vi "Main.vi"() -> ()   [LabVIEW 2017]
uses:
  logo.ctl
  <vilib>/Utility/error.llb/DialogType.ctl
  <userlib>/SimuLabAPIEx_V3/SimuLabAPIEx_V3.lvlib
panel:
  out "剩余日志条数":i32
  out "function return 2":i32
  out "nStatus out":i32
  out "注册参数瞬态返回值":i32
  in  "信号1":i32(listbox)
  out "方法返回值":i32
  in  "注销录制组":bool
  in  "录制组名称":string
  out "录制组状态":i32
  out "方法返回值":i32
  in  "获取录制组状态":bool
  in  "录制组名称":string
  in  "列表长度":i32
  out "方法返回值":i32
  out "返回信号ID":i32
  in  "获取信号ID通过名称":bool
  in  "信号名称":string
  out "function return":i32
  out "nOutSigParamOffsetList out":i32[](array[numeric])
  out "nOutSigParamIdList out":i32[](array[numeric])
  in  "注册录制组":bool
  in  "参数输出信号偏移":i32[](array[numeric])
  in  "参数/输出信号ID列表":i32[](array[numeric])
  in  "录制文件名":string
  in  "存储文件的路径":string
  in  "数据格式":i32
  in  "录制时长":dbl
  in  "采样率":i32
  in  "录制组名称":string
  out "信号连续返回值":dbl[](array[numeric])
  out "pTimeOffset out":dbl[](array[numeric])
  out "实际有效数据长度":i32
  out "信连方法返回值":i32
  in  "获取信号值连续":bool
  in  "数组偏移":i32
  in  "信号名称":string
  out "返回的信号值":dbl[](array[numeric])
  out "实际有效数据长度":i32
  out "时间偏移返回值":dbl
  out "信瞬方法返回值":i32
  in  "获取信号值瞬态":bool
  in  "数组偏移":i32
  in  "信号名称":string
  out "方法返回值":i32
  out "返回的日志级别":i32
  out "返回的日志信息":string
  out "返回的时间偏移":dbl[](array[numeric])
  out "返回的参数值":dbl[](array[numeric])
  out "实际有效数据长度":i32
  out "获取参数值连续返回值":i32
  in  "获取参数值连续":bool
  in  "数组偏移":i32
  in  "参数名称":string
  out "实际有效数据长度":i32
  out "时间偏移返回值":dbl
  out "pDataValue out":dbl[](array[numeric])
  out "获取参数值瞬态返回值":i32
  in  "获取参数值瞬态":bool
  in  "数组偏移":i32
  in  "参数名称":string
  out "注销输出信号连续返回值":i32
  in  "注销输出信号连续":bool
  in  "数组偏移":i32
  in  "输出信号名称":string
  out "注册输出信号连续返回值":i32
  in  "注册输出信号连续":bool
  in  "数组偏移":i32
  in  "输出信号名称":string
  out "注销输出信号瞬态返回值":i32
  in  "注销输出信号瞬态":bool
  in  "数组偏移":i32
  in  "输出信号名称":string
  out "注册输出信号瞬态返回值":i32
  in  "注册输出信号瞬态":bool
  in  "数组偏移":i32
  in  "输出信号名称":string
  out "pData":dbl[](array[numeric])
  out "方法返回值":i32
  in  "获取参数值":bool
  in  "数组偏移量":i32
  in  "参数名称":string
  out "注销连续返回值":i32
  in  "注销连续":bool
  in  "数组偏移":i32
  in  "参数名称":string
  out "注册参数连续返回值":i32
  in  "注册参数连续":bool
  in  "数组偏移":i32
  in  "参数名称":string
  out "注销参数瞬态返回值":i32
  in  "注销参数瞬态":bool
  in  "数组偏移":i32
  in  "参数名称":string
  in  "数组偏移":i32
  in  "注册参数瞬态":bool
  in  "参数名称":string
  in  "数组偏移量":i32
  out "pData":dbl[](array[numeric])
  out "方法返回值":i32
  in  "获取信号值":bool
  in  "信号名称":string
  out "方法返回值":i32
  out "模型名称":string
  in  "根据参数名称获取模型名称":bool
  in  "参数名称":string
  out "方法返回值":i32
  out "返回参数ID":i32
  in  "获取参数ID通过名称":bool
  in  "参数名称":string
  out "方法返回值":i32
  out "返回模型ID":i32
  in  "模型名称获取ID":bool
  in  "模型名称":string
  out "返回的下位机IP":string
  in  "模型的下位机IP":bool
  in  "模型名称":string
  out "方法返回值":i32
  out "返回的模型信息":string
  in  "获取指定模型序号模型信息":bool
  in  "模型序号":i32
  out "参数个数":i32
  in  "获取参数个数":bool
  out "模型个数":i32
  in  "获取模型个数":bool
  in  "获取仿真系统日志信息":bool
  out "dMoniData":dbl[](array[numeric])
  out "超时返回值":i32
  out "方法返回值":i32
  in  "获取模型仿真状态":bool
  in  "模型名称输入框":string
  out "方法返回值":i32
  out "状态返回值":i32
  in  "获取工程状态":bool
  out "方法返回值":i32
  out "返回的错误信息":string
  in  "获取最后错误信息":bool
  in  "缓冲点数":i32=20000
  in  "参数索引（1-N）":i32=1 min=1
  in  "缓冲示波个数":i32=10000
  in  "列表已更新":bool=TRUE
  in  "刷新图形":bool
  out "XY Graph":T1(graph)={"pTimeOffset out"=[747.164, 747.165, 747.166, 747.167, 747.168, 747.169, 747.17, 747.171, 747.172, 747.173, 747.174, 747.1750000000001, 747.176, 747.177, 747.178, 747.179, 747.1800000000001, 747.181, 747.182, 747.183, 747.184, 747.1850000000001, 747.186, 747.187, 747.188, 747.189, 747.19, 747.191, 747.192, 747.193, 747.194, 747.195, 747.196, 747.197, 747.198, 747.1990000000001, 747.2, 747.201, 747.202, 747.203, 747.2040000000001, 747.205, 747.206, 747.207, 747.208, 747.2090000000001, 747.21, 747.211, 747.212, 747.213, 747.214, 747.215, 747.216, 747.217, 747.218, 747.219, 747.22, 747.221, 747.222, 747.2230000000001, 747.224, 747.225, 747.226, 747.227, 747.2280000000001, 747.229, 747.23, 747.231, 747.232, 747.2330000000001, 747.234, 747.235, 747.236, 747.237, 747.238, 747.239, 747.24, 747.241, 747.242, 747.243, 747.244, 747.245, 747.246, 747.2470000000001, 747.248, 747.249, 747.25, 747.251, 747.2520000000001, 747.253, 747.254, 747.255, 747.256, 747.2570000000001, 747.258, 747.259, 747.26, 747.261, 747.2620000000001, 747.263, 747.264, 747.265, 747.266, 747.267, 747.268, 747.269, 747.27, 747.2710000000001, 747.272, 747.273, 747.274, 747.275, 747.2760000000001, 747.277, 747.278, 747.279, 747.28, 747.2810000000001, 747.282, 747.283, 747.284, 747.285, 747.2860000000001, 747.287, 747.288, 747.289, 747.29, 747.291, 747.292, 747.293, 747.294, 747.295, 747.296, 747.297, 747.298, 747.299, 747.3000000000001, 747.301, 747.302, 747.303, 747.304, 747.3050000000001, 747.306, 747.307, 747.308, 747.309, 747.3100000000001, 747.311, 747.312, 747.313, 747.314, 747.315, 747.316, 747.317, 747.318, 747.319, 747.32, 747.321, 747.322, 747.323, 747.3240000000001, 747.325, 747.326, 747.327, 747.328, 747.3290000000001, 747.33, 747.331, 747.332, 747.333, 747.3340000000001, 747.335, 747.336, 747.337, 747.338, 747.339, 747.34, 747.341, 747.342, 747.343, 747.344, 747.345, 747.346, 747.347, 747.3480000000001, 747.349, 747.35, 747.351, 747.352, 747.3530000000001, 747.354, 747.355, 747.356, 747.357, 747.3580000000001, 747.359, 747.36, 747.361, 747.362, 747.363, 747.364, 747.365, 747.366, 747.367, 747.368, 747.369, 747.37, 747.371, 747.3720000000001, 747.373, 747.374, 747.375], "pDataValue out"=[-0.5107453766165692, -0.509885389359039, -0.5090248922161622, -0.5081638860483376, -0.5073023717167672, -0.5064403500828674, -0.5055778220086596, -0.5047147883566722, -0.5038512499898401, -0.5029872077718983, -0.5021226625667906, -0.5012576152390622, -0.500392066653662, -0.4995260176763352, -0.49865946917303233, -0.49779242201030194, -0.496924877055191, -0.4960568351751457, -0.4951882972384053, -0.49431926411340893, -0.4934497366691897, -0.4925797157752749, -0.4917092023015864, -0.49083819711883553, -0.4899667010979285, -0.4890947151103612, -0.4882222400281196, -0.48734927672357936, -0.48647582606990225, -0.48560188894043965, -0.48472746620912865, -0.4838525587503918, -0.482977167439037, -0.48210129315065453, -0.48122493676101913, -0.4803480991464871, -0.47947078118379616, -0.4785929837504638, -0.4777147077241875, -0.47683595398324335, -0.475956723406385, -0.47507701687274284, -0.47419683526222345, -0.47331617945490834, -0.4724350503314532, -0.47155344877298716, -0.4706713756610113, -0.46978883187779935, -0.46890581830579464, -0.4680223358280108, -0.46713838532793006, -0.4662539676894024, -0.46536908379704645, -0.4644837345356455, -0.4635979207905488, -0.4627116434475699, -0.46182490339288534, -0.46093770151343666, -0.4600500386963249, -0.4591619158292128, -0.4582733338001221, -0.45738429349783677, -0.45649479581129615, -0.45560484162999776, -0.4547144318438957, -0.45382356734329843, -0.4529322490192729, -0.45204047776303613, -0.4511482544663593, -0.4502555800214656, -0.44936245532092783, -0.44846888125807377, -0.4475748587263758, -0.4466803886198565, -0.4457854718329857, -0.44489010926057854, -0.44399430179820093, -0.4430980503415586, -0.4422013557869028, -0.4413042190309281, -0.44040664097066906, -0.4395086225039079, -0.4386101645285608, -0.43771126794308574, -0.43681193364627696, -0.4359121625376732, -0.43501195551694327, -0.43411131348429405, -0.43321023734036757, -0.43230872798613734, -0.43140678632331764, -0.4305044132537476, -0.42960160967980016, -0.4286983765042789, -0.42779471463031415, -0.4268906249617731, -0.42598610840264267, -0.4250811658574394, -0.4241757982311057, -0.42327000642890616, -0.4223637913568384, -0.4214571539210145, -0.42055009502807184, -0.4196426155850692, -0.41873471649938276, -0.4178263986791179, -0.41691766303248917, -0.41600851046823223, -0.41509894189539603, -0.41418895822375595, -0.4132785603631922, -0.4123677492241025, -0.411456525717298, -0.41054489075389844, -0.40963284524574595, -0.40872039010478234, -0.4078075262434627, -0.4068942545746509, -0.4059805760115145, -0.4050664914679398, -0.4041520018579074, -0.40323710809590685, -0.40232181109683185, -0.40140611177587515, -0.4004900110489442, -0.3995735098320356, -0.3986566090416505, -0.3977393095946896, -0.3968216124083479, -0.39590351840053123, -0.3949850284892291, -0.39406614359293146, -0.3931468646305231, -0.39222719252117827, -0.3913071281847782, -0.39038667254128256, -0.3894658265111469, -0.38854459101511246, -0.3876229669746241, -0.38670095531120113, -0.3857785569468551, -0.38485577280398425, -0.3839326038052677, -0.3830090508740843, -0.382085114933882, -0.38116079690859656, -0.380236097722546, -0.37931101830032427, -0.37838555956722103, -0.3774597224485897, -0.37653350787026746, -0.37560691675846875, -0.37467995003967913, -0.3737526086410761, -0.3728248934898956, -0.37189680551385274, -0.3709683456410353, -0.3700395147997976, -0.3691103139191815, -0.36818074392828226, -0.3672508057566698, -0.3663205003341764, -0.36538982859131897, -0.3644587914586634, -0.36352738986724675, -0.36259562474847057, -0.36166349703399386, -0.36073100765615623, -0.359798157547341, -0.3588649476403983, -0.3579313788685378, -0.3569974521652221, -0.3560631684645902, -0.35512852870081946, -0.3541935338085497, -0.3532581847227756, -0.35232248237873987, -0.3513864277123575, -0.35045002165957667, -0.3495132651568035, -0.3485761591407942, -0.3476387045485483, -0.3467009023177334, -0.345762753386045, -0.34482425869163214, -0.3438854191728825, -0.34294623576884914, -0.3420067094186086, -0.34106684106168716, -0.3401266316379531, -0.3391860820875088, -0.33824519335111763, -0.3373039663695613, -0.3363624020840667, -0.33542050143619806, -0.33447826536774883, -0.33353569482116924, -0.3325927907389226, -0.33164955406391294, -0.33070598573937693, -0.3297620867087754, -0.3288178579162219, -0.327873300305838, -0.32692841482218105, -0.32598320241013656, -0.3250376640148094, -0.3240918005819527, -0.3231456130573225, -0.32219910238710614, -0.32125226951770663, -0.320305115396172, -0.31935764096954866]} caption="信号波形图"
  in  "工程配置文件":path=path "C:/testProj/testProj/main.slm"
  out "加载状态":bool
  out "加载返回值":i32 caption="返回值"
  in  "参数":i32(listbox)=-1
  in  "信号":i32(listbox)=2
  in  "重置":bool
  in  "暂停":bool
  in  "开始":bool
  in  "加载":bool
  in  "logo":T2
  in  "退出":bool
  out "连接状态":bool=TRUE
  out "连接返回值":i32 caption="返回值"
  in  "仿真系统上位机IP地址":string="192.168.1.52"
  in  "连接":bool
  # "Simulab 仿 真 测 试 平 台 演 示 Demo V3.0"
  # "双击参数进行调参"
  # "双击信号图形显示"
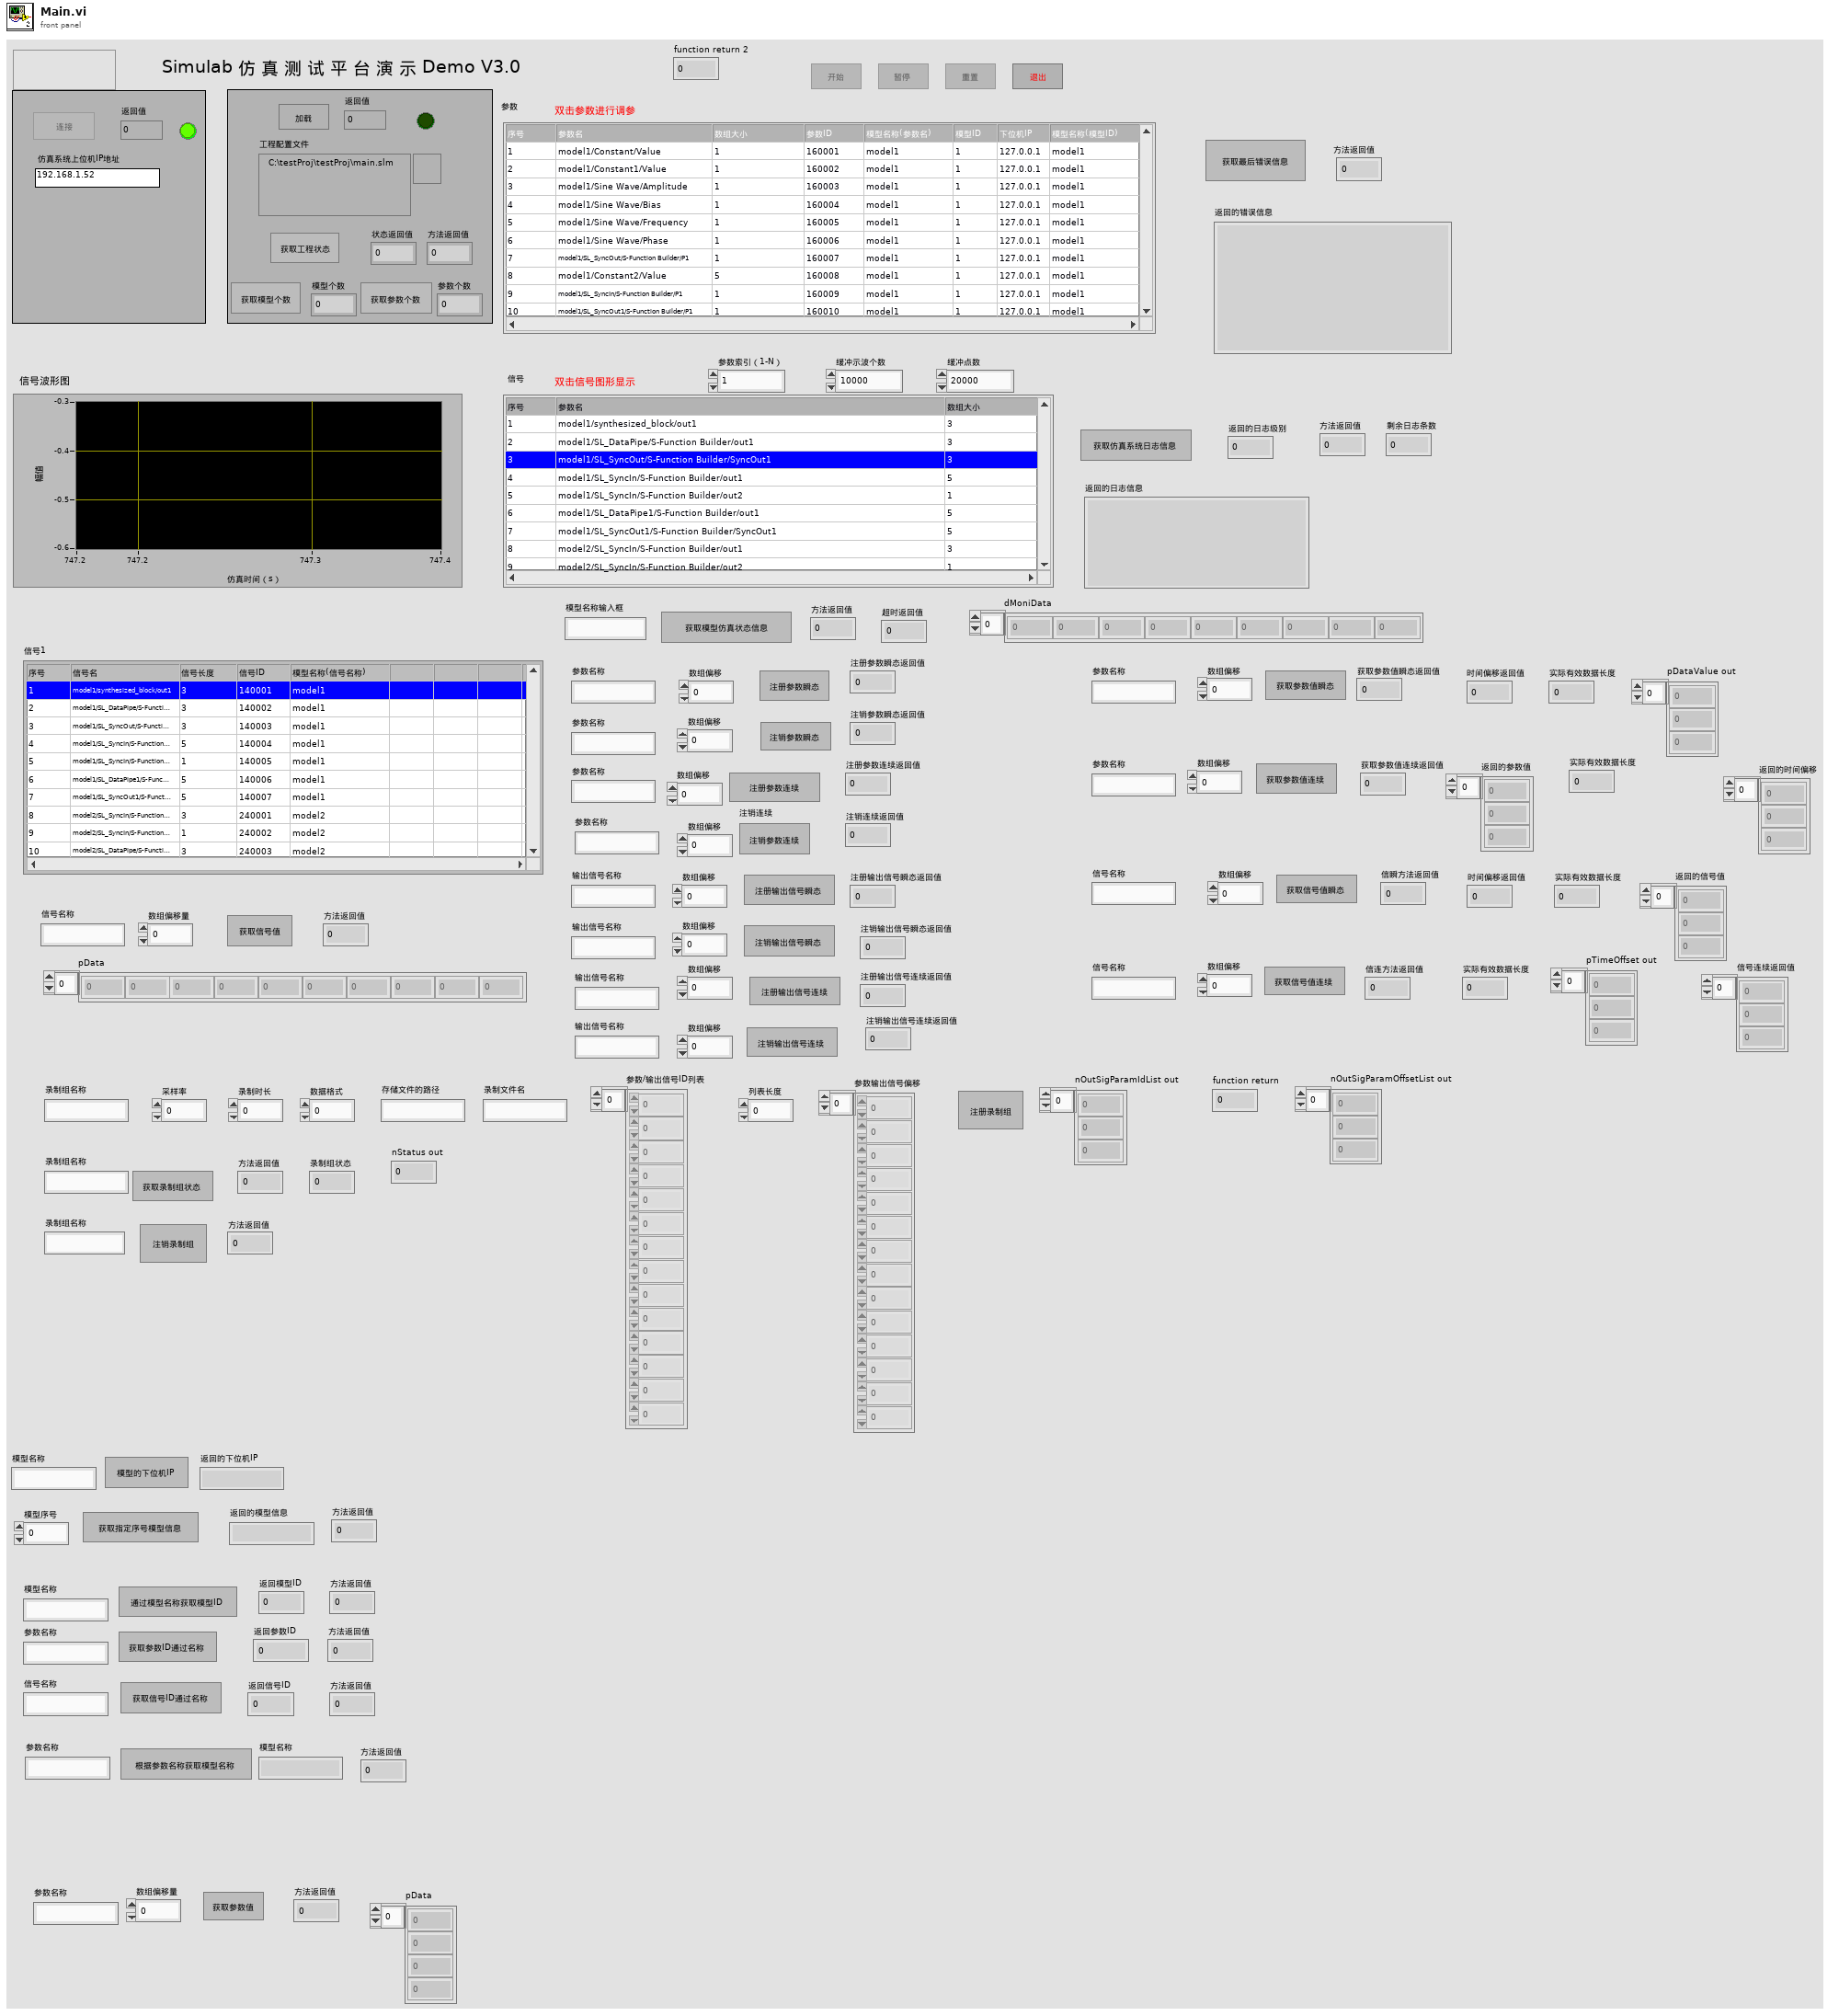
[diagram p1: front panel]
types:
  T1 = cluster{"pTimeOffset out":dbl[], "pDataValue out":dbl[]}
  T2 = typedef "logo.ctl" = bool
  T3 = enum16{"idle", "initial", "connect target", "load project", "get state", "monitoring", "exit", "error"}
  T4 = enum8{"Enabled", "Disabled", "Disabled and Grayed Out"}
  T5 = enum8{"Enabled", "Disabled", "Disabled and Grayed Out"}[]
  T6 = typedef "DialogType.ctl" = u16
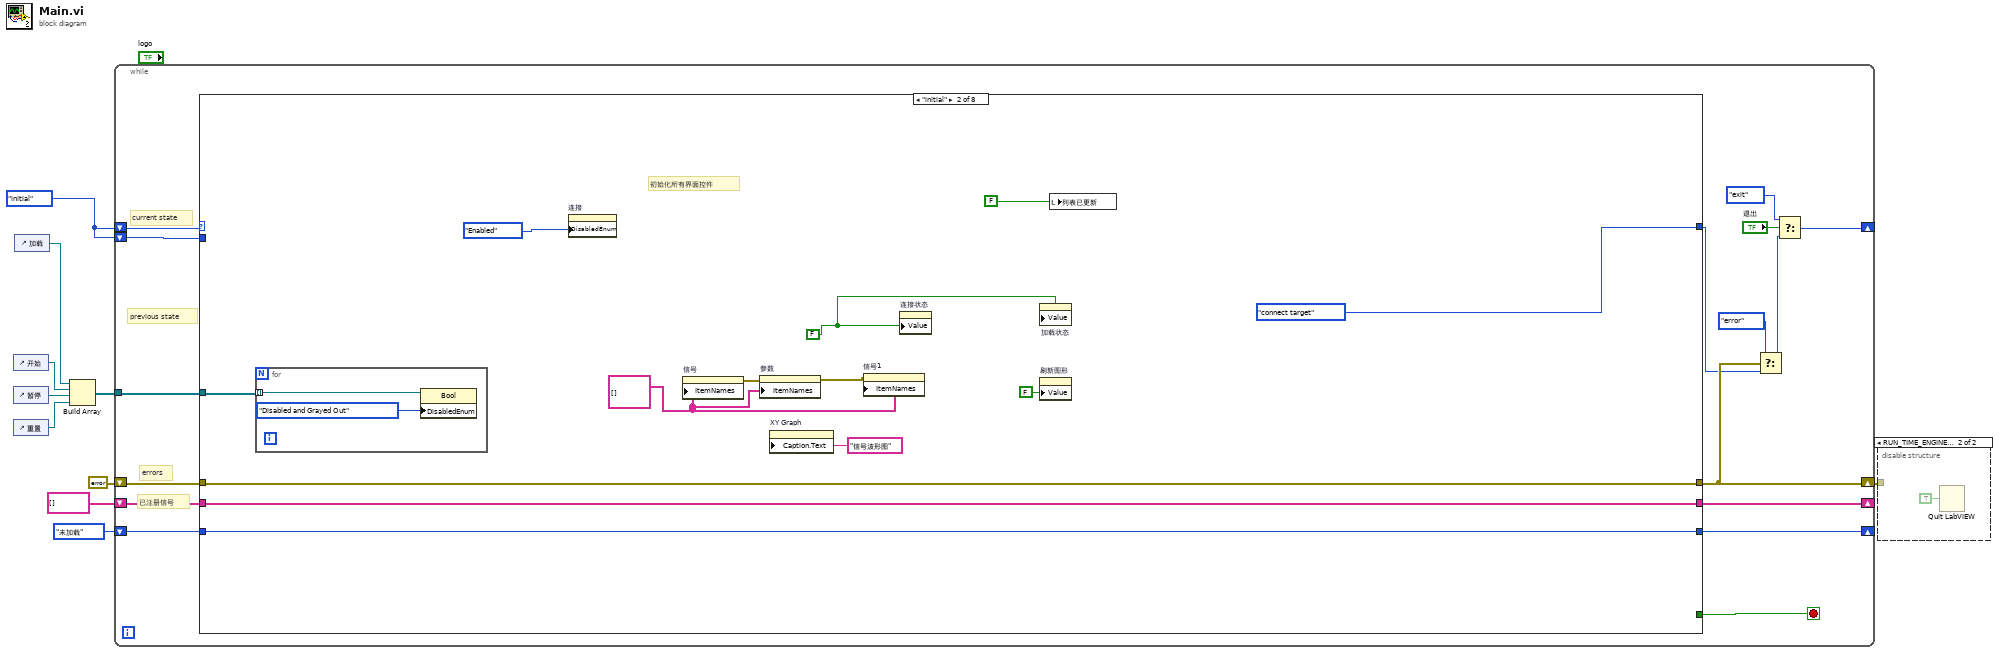
[diagram p0: block diagram]
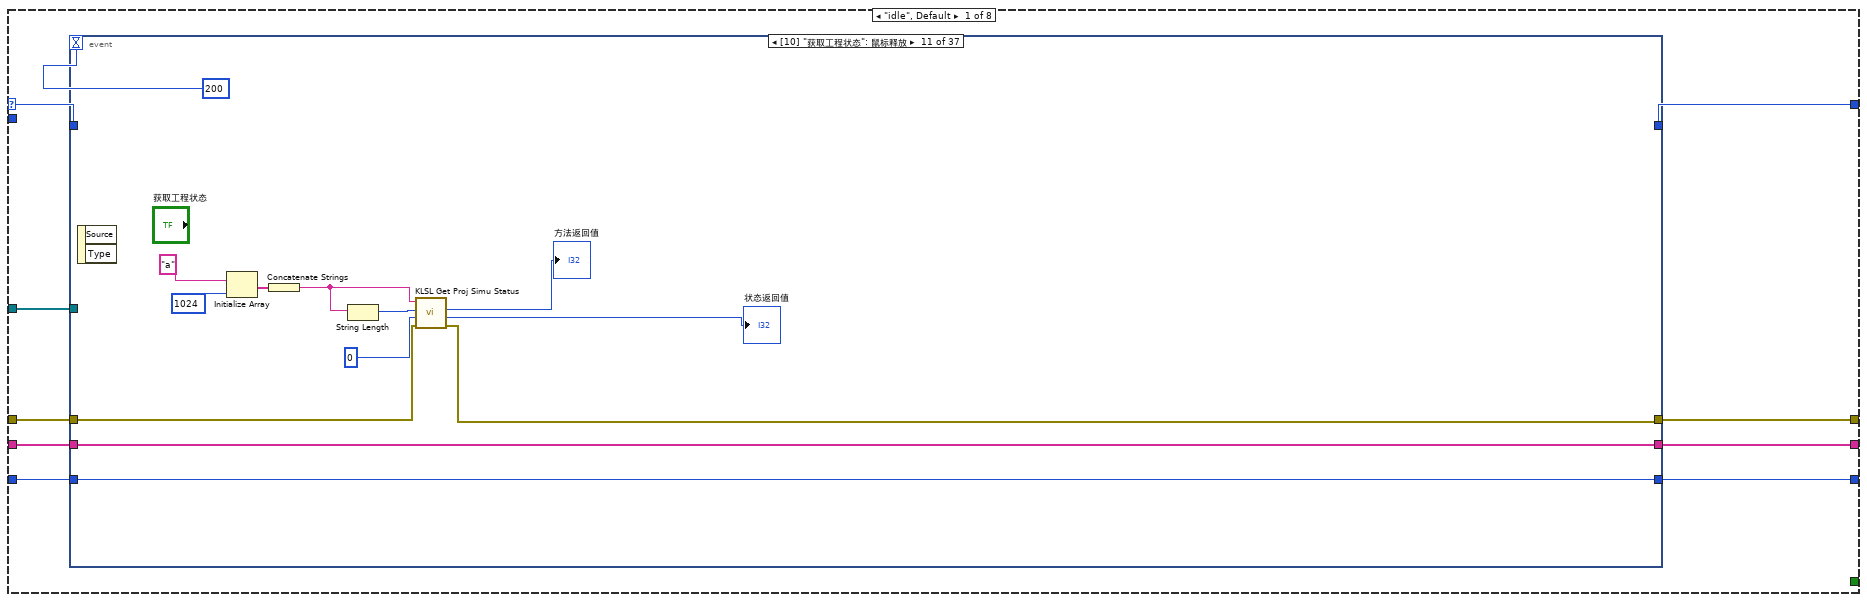
[diagram p3: hidden frame]
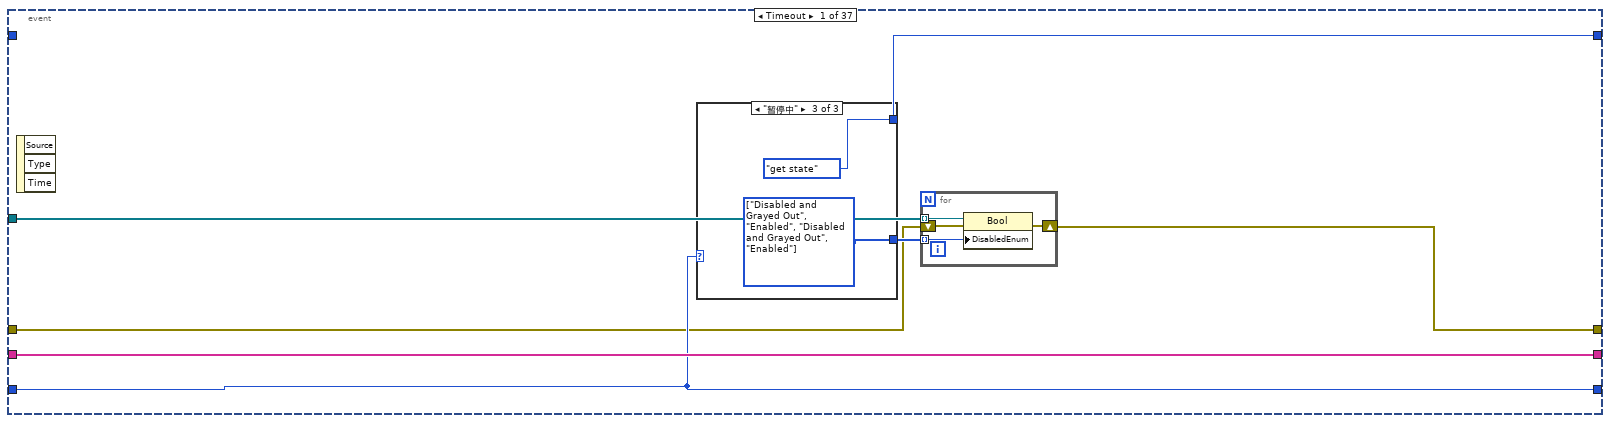
[diagram p4: hidden frame]
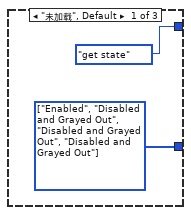
[diagram p5: hidden frame]
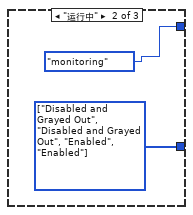
[diagram p6: hidden frame]
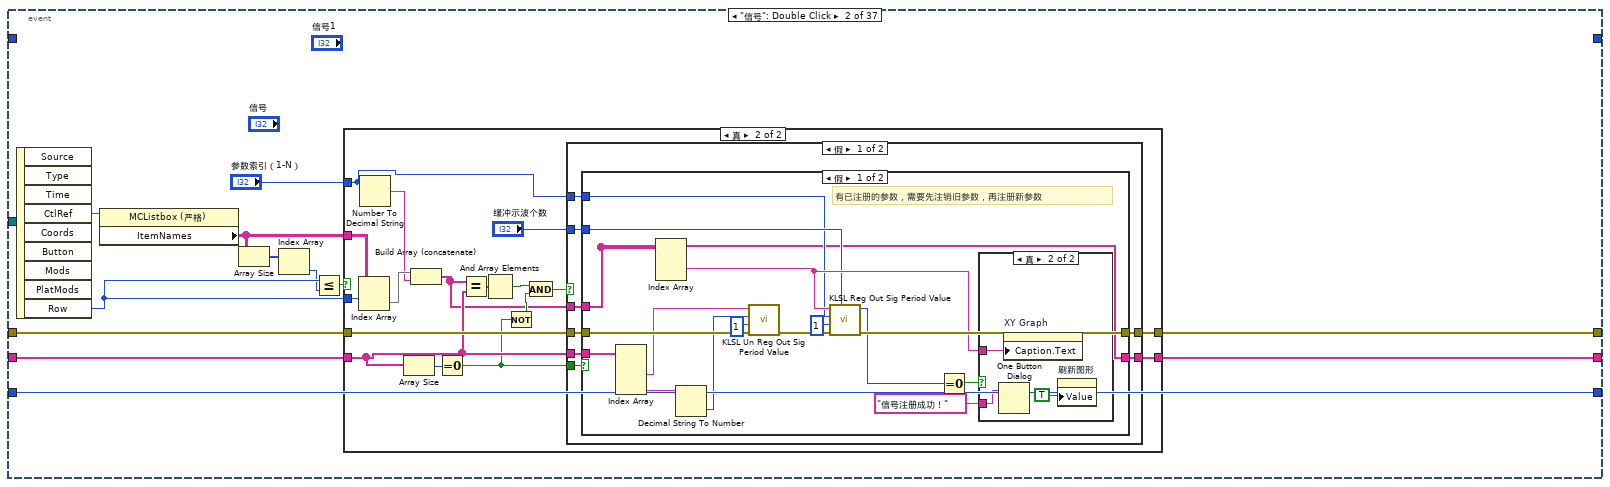
[diagram p7: hidden frame]
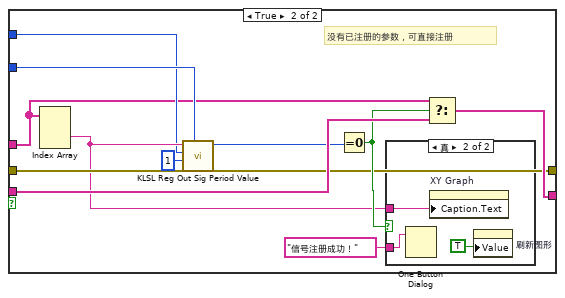
[diagram p10: hidden frame]
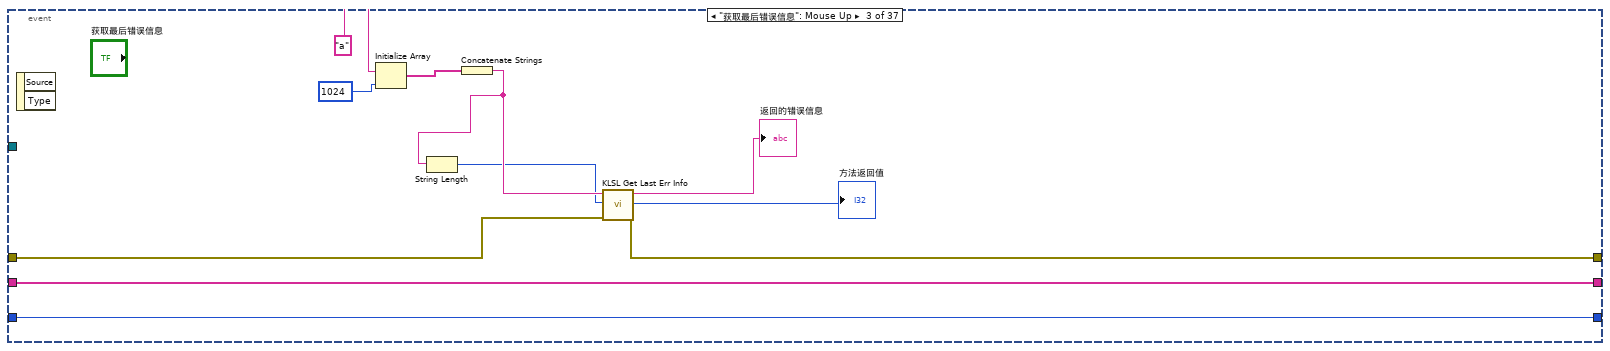
[diagram p13: hidden frame]
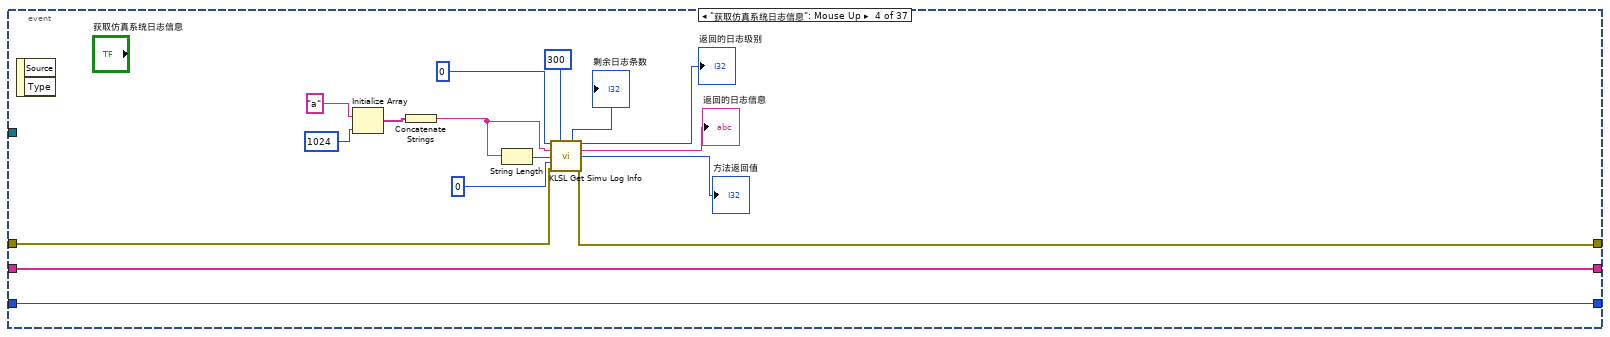
[diagram p14: hidden frame]
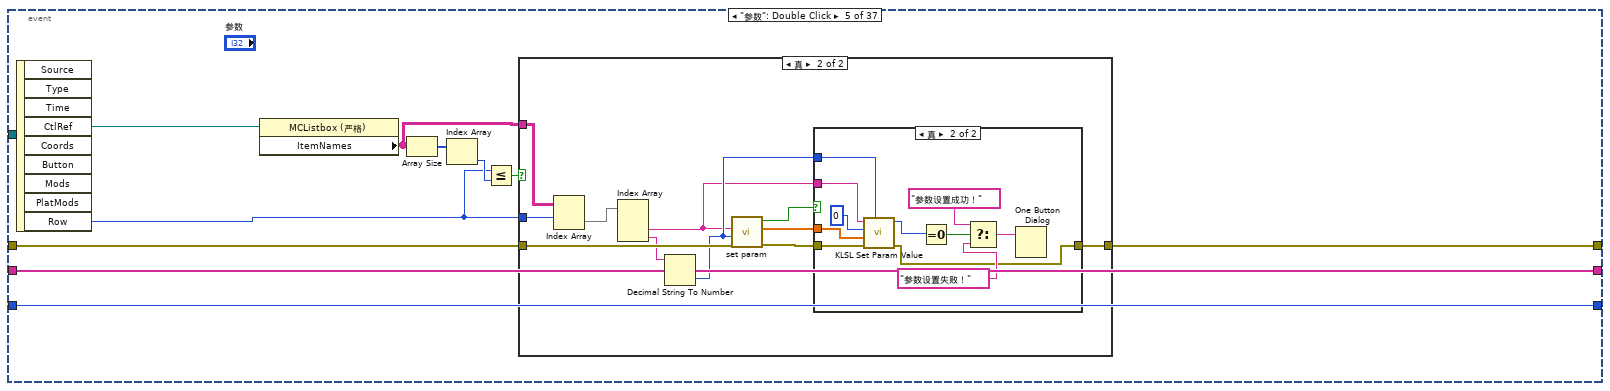
[diagram p15: hidden frame]
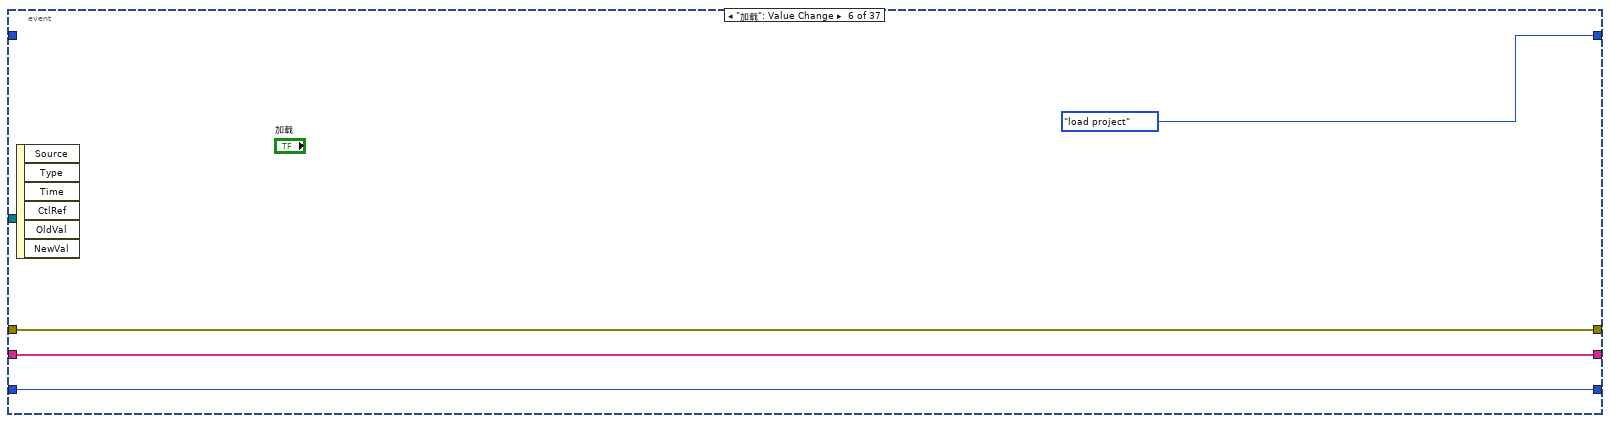
[diagram p18: hidden frame]
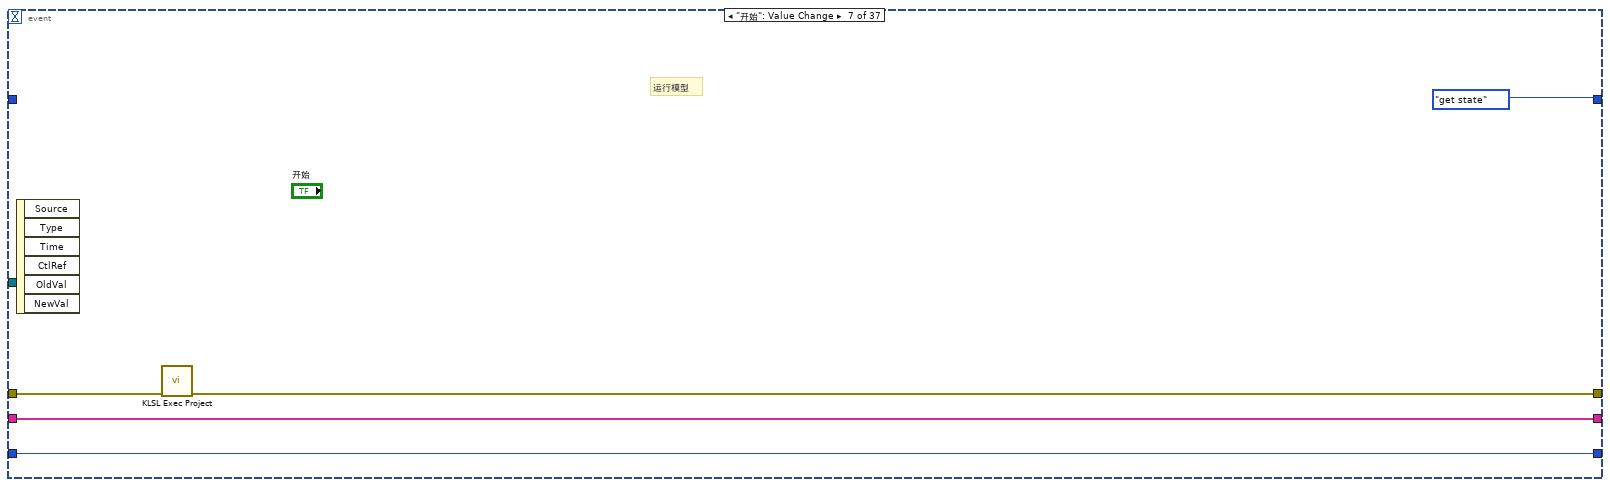
[diagram p19: hidden frame]
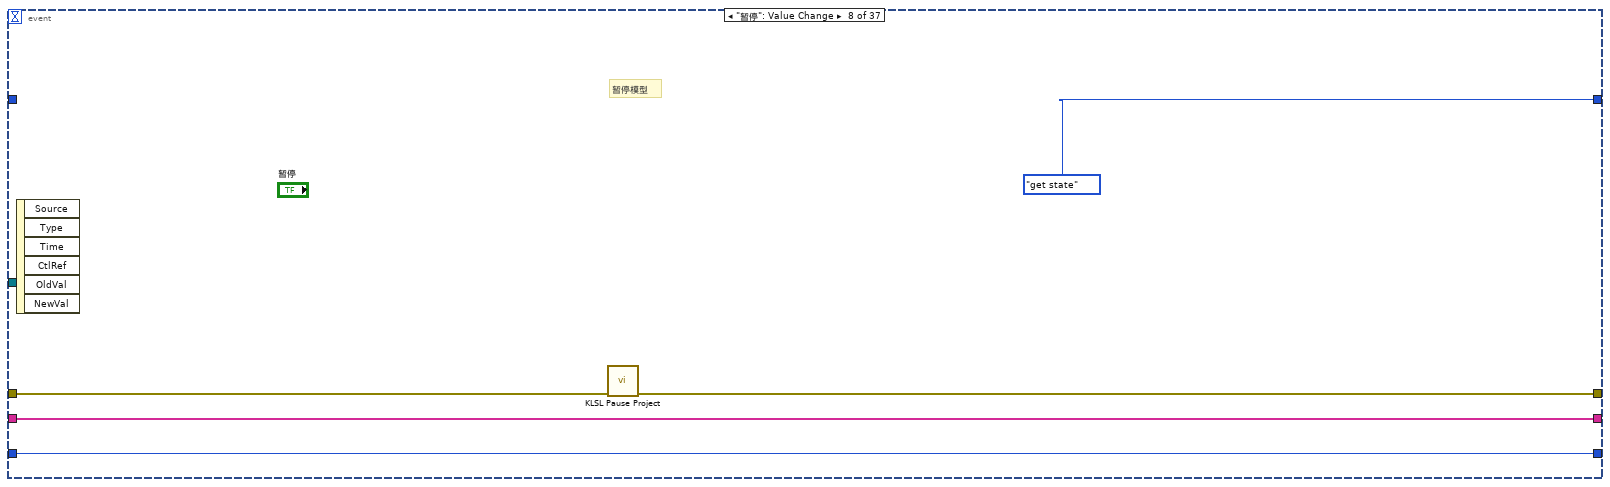
[diagram p20: hidden frame]
diagram:
  w1 = T3."initial"
  n1 = control-ref of="开始"() -> (w8:refnum<vi>)
  n2 = control-ref of="暂停"() -> (w7:refnum<vi>)
  n3 = control-ref of="重置"() -> (w6:refnum<vi>)
  n4 = control-ref of="加载"() -> (w4:refnum<vi>)
  n5 = Build Array(w4, w8, w7, w6) -> (w9:refnum<vi>[])
  n6 = while {
    shift-right: [w16] -> _
    shift-left: w1 -> [w26]
    shift-right: [w21] -> w2
    shift-left: errorcluster {"status"=FALSE, "code"=0, "source"=""} ("错误常量") -> [w25]
    shift-left: w1 -> [w24]
    shift-right: [w13] -> _
    shift-left: enum16{"未加载", "运行中", "暂停中"}."未加载" -> [w18]
    tunnel: w9 -> [w17]
    shift-right: [w14] -> _
    shift-left: string[] [] ("信号 2") -> [w15]
    stop <- w23 stop-if-true
    # "已注册信号"
    # "errors"
    # "previous state"
    # "current state"
    n7 = case shown="\"initial\"" w26 {
      selector: w26 -> [w32 _ _ _ _ _ _ _]
      tunnel: w25 -> [w35 w510 w520 w534 w565 w582 w618 w627]
      tunnel: [w34 w510 w513 w531 w563 w574 w617 w625] -> w21
      tunnel: [w31 T3."connect target" w517 T3."idle" T3."get state" T3."get state" T3."exit" _] -> w20
      tunnel: w24 -> [_ _ _ _ _ _ _ _]
      tunnel: [_ _ _ _ _ _ TRUE _] -> w23
      tunnel: w18 -> [w33 w505 w516 w540 w569 w576 w620 w623]
      tunnel: w17 -> [w29 w509 _ _ _ _ _ _]
      tunnel: w15 -> [w30 w507 w519 w541 w570 w578 w621 w624]
      tunnel: [w28 w507 w519 w541 w570 w577 w621 w624] -> w14
      tunnel: [w27 w505 w516 w533 w569 w576 w620 w623] -> w13
      frame "idle", Default {
        n8 = event shown="[10] \"获取工程状态\": 鼠标释放" {
          selector: _ -> [_ _ _ _ _ _ _ _ _ _ _ _ _ _ _ _ _ _ _ _ _ _ _ _ _ _ _ _ _ _ _ _ _ _ _ _ _]
          dyn-events: _ -> [_ _ _ _ _ _ _ _ _ _ _ _ _ _ _ _ _ _ _ _ _ _ _ _ _ _ _ _ _ _ _ _ _ _ _ _ _]
          timeout: 200 -> [_ _ _ _ _ _ _ _ _ _ _ _ _ _ _ _ _ _ _ _ _ _ _ _ _ _ _ _ _ _ _ _ _ _ _ _ _]
          tunnel: w35 -> [w37 w64 w137 w153 w157 w191 w195 w200 w209 w215 w226 w239 w245 w251 w263 w274 w282 w290 w302 w313 w319 w335 w350 w357 w366 w374 w385 w392 w407 w414 w423 w438 w446 w463 w481 w487 w495]
          tunnel: [w39 w63 w136 w152 w156 w191 w194 w199 w210 w215 w225 w238 w244 w250 w262 w273 w281 w289 w301 w312 w317 w334 w349 w356 w365 w373 w384 w391 w406 w413 w422 w437 w445 w450 w480 w486 w494] -> w34
          tunnel: w33 -> [w38 w65 w139 w155 w163 w193 w198 w203 w212 w216 w228 w241 w247 w253 w265 w276 w284 w292 w304 w315 w322 w337 w352 w359 w367 w376 w387 w394 w409 w416 w425 w440 w448 w465 w483 w489 w497]
          tunnel: w32 -> [_ _ _ _ _ _ _ _ _ _ _ _ _ _ _ _ _ _ _ _ _ _ _ _ _ _ _ _ _ _ _ _ _ _ _ _ _]
          tunnel: [w43 _ _ _ _ T3."load project" T3."get state" T3."get state" T3."get state" T3."exit" _ _ _ _ _ _ _ _ _ _ _ _ _ _ _ _ _ _ _ _ _ _ _ _ _ _ _] -> w31
          tunnel: w30 -> [w42 w61 w138 w154 w164 w192 w197 w202 w204 w214 w227 w240 w246 w252 w264 w275 w283 w291 w303 w314 w321 w336 w351 w358 w368 w375 w386 w393 w408 w415 w424 w439 w447 w464 w482 w488 w496]
          tunnel: w29 -> [w41 _ _ _ _ _ _ _ _ _ _ _ _ _ _ _ _ _ _ _ _ _ _ _ _ _ _ _ _ _ _ _ _ _ _ _ _]
          tunnel: [w42 w62 w138 w154 w164 w192 w197 w202 w206 w214 w227 w240 w246 w252 w264 w275 w283 w291 w303 w314 w321 w336 w351 w358 w368 w375 w386 w393 w408 w415 w424 w439 w447 w464 w482 w488 w496] -> w28
          tunnel: [w38 w65 w139 w155 w163 w193 w198 w203 w212 w216 w228 w241 w247 w253 w265 w276 w284 w292 w304 w315 w322 w337 w352 w359 w367 w376 w387 w394 w409 w416 w425 w440 w448 w465 w483 w489 w497] -> w27
          event Timeout {
            n9 = event-data() -> ()  [unwired: 1 in, 3 out]
            n10 = case shown="\"暂停中\"" w38 {
              tunnel: [T3."get state" T3."monitoring" T3."get state"] -> w43
              tunnel: [w49 w51 w53] -> w40
              frame "未加载", Default {
                w49 = T5 [enum."Enabled", enum."Disabled and Grayed Out", enum."Disabled and Grayed Out", enum."Disabled and Grayed Out"] items=["Enabled", "Disabled", "Disabled and Grayed Out"]
              }
              frame "运行中" {
                w51 = T5 [enum."Disabled and Grayed Out", enum."Disabled and Grayed Out", enum."Enabled", enum."Enabled"] items=["Enabled", "Disabled", "Disabled and Grayed Out"]
              }
              frame "暂停中" {
                w53 = T5 [enum."Disabled and Grayed Out", enum."Enabled", enum."Disabled and Grayed Out", enum."Enabled"] items=["Enabled", "Disabled", "Disabled and Grayed Out"]
              }
            }
            n11 = for {
              tunnel: w41 -> [w47] mode=indexing
              tunnel: w40 -> [w46] mode=indexing
              shift-right: [w44] -> w39
              shift-left: w37 -> [w45]
              n12 = property class="Bool"(reference=w47, error in=w45, "DisabledEnum"=w46) -> (error out=w44:errorcluster)  [unwired: 1 out]
            }
          }
          event "信号": Double Click {
            n13 = event-data() -> ("CtlRef"=w60:refnum<vi>, "Row"=w57:i32)  [unwired: 1 in, 7 out]
            n14 = property class="MCListbox (严格)"(reference=w60) -> ("ItemNames"=w59:string[][])  [unwired: 1 in, 2 out]
            n15 = Array Size(array=w59) -> (size(s)=w58:i32[])
            n16 = Index Array(array=w58) -> (element=w56:i32)  [unwired: 1 in]
            n17 = Less Or Equal?(x=w57, y=w56) -> (x <= y?=w55:bool)
            n18 = case shown="真" w55 {
              tunnel: w64 -> [w67 w84]
              tunnel: [w67 w83] -> w63
              tunnel: [w66 w81] -> w62
              tunnel: w61 -> [w66 w80]
              tunnel: w59 -> [_ w78]
              tunnel: w57 -> [_ w77]
              tunnel: "参数索引（1-N）" -> [_ w68]
              frame False {
              }
              frame True {
                n19 = Index Array(array=w78, index (row)=w77) -> (element=w71:string[])  [unwired: 1 in]
                n20 = Number To Decimal String(number=w68) -> (decimal integer string=w69:string)  [unwired: 1 in]
                n21 = Array Size(array=w80) -> (size(s)=w82:i32)
                n22 = Build Array (concatenate)(w71, w69) -> (w70:string[])
                n23 = Equal To 0?(x=w82) -> (x = 0?=w73:bool)
                n24 = Equal?(x=w70, y=w80) -> (x = y?=w79:bool[])
                n25 = And Array Elements(Boolean array=w79) -> (logical AND=w76:bool)
                n26 = Not(x=w73) -> (.not. x?=w74:bool)
                n27 = And(x=w76, y=w74) -> (x .and. y?=w75:bool)
                n28 = case shown="假" w75 {
                  tunnel: w84 -> [w92 w128]
                  tunnel: [w91 w128] -> w83
                  tunnel: w73 -> [w90 _]
                  tunnel: [w89 w127] -> w81
                  tunnel: w80 -> [w88 w127]
                  tunnel: w70 -> [w87 _]
                  tunnel: "缓冲示波个数" -> [w86 _]
                  tunnel: w68 -> [w85 _]
                  frame False {
                    n29 = case shown="假" w90 {
                      tunnel: w92 -> [w105 w119]
                      tunnel: [w102 w118] -> w91
                      tunnel: w87 -> [w94 w112]
                      tunnel: w88 -> [w108 w123]
                      tunnel: [w94 w122] -> w89
                      tunnel: w86 -> [w99 w115]
                      tunnel: w85 -> [w95 w113]
                      frame False {
                        # "有已注册的参数，需要先注销旧参数，再注册新参数"
                        n30 = Index Array(array=w108) -> (element #2=w104:string, element #4=w98:string)  [unwired: 4 in, 2 out]
                        n31 = Index Array(array=w94) -> (element #2=w100:string)  [unwired: 3 in, 2 out]
                        n32 = Decimal String To Number(string=w98) -> (number=w97:i32)  [unwired: 2 in, 1 out]
                        n33 = call <userlib>:"KLSL Un Reg Out Sig Period Value.vi"("error in (no error)"=w105, "nSampleUs"=1, "nOffSet"=w97, "szOutSigName"=w104) -> ("error out"=w103:errorcluster)  [unwired: 6 in, 1 out]
                        n34 = call <userlib>:"KLSL Reg Out Sig Period Value.vi"("nCachedDataCount"=w99, "error in (no error)"=w103, "nSampleUs"=1, "nOffSet"=w95, "szOutSigName"=w100) -> ("error out"=w102:errorcluster, "function return"=w101:i32)  [unwired: 5 in]
                        n35 = Equal To 0?(x=w101) -> (x = 0?=w107:bool)
                        n36 = case shown="真" w107 {
                          tunnel: "信号注册成功！" -> [_ w111]
                          tunnel: w100 -> [_ w109]
                          frame False {
                          }
                          frame True {
                            n37 = One Button Dialog(message=w111) -> ()  [unwired: 1 in, 1 out]
                            n38 = property on="XY Graph" class="XYGraph (严格)"("Caption.Text"=w109) -> ()  [unwired: 2 in, 2 out]
                            n39 = property on="刷新图形" class="Bool (严格)"("Value"=TRUE ("刷新图形")) -> ()  [unwired: 2 in, 2 out]
                          }
                        }
                      }
                      frame True {
                        # "没有已注册的参数，可直接注册"
                        n40 = Index Array(array=w112) -> (element #2=w117:string)  [unwired: 3 in, 2 out]
                        n41 = call <userlib>:"KLSL Reg Out Sig Period Value.vi"("nCachedDataCount"=w115, "error in (no error)"=w119, "nSampleUs"=1, "nOffSet"=w113, "szOutSigName"=w117) -> ("error out"=w118:errorcluster, "function return"=w116:i32)  [unwired: 5 in]
                        n42 = Equal To 0?(x=w116) -> (x = 0?=w121:bool)
                        n43 = case shown="真" w121 {
                          tunnel: "信号注册成功！" -> [_ w126]
                          tunnel: w117 -> [_ w124]
                          frame False {
                          }
                          frame True {
                            n44 = One Button Dialog(message=w126) -> ()  [unwired: 1 in, 1 out]
                            n45 = property on="XY Graph" class="XYGraph (严格)"("Caption.Text"=w124) -> ()  [unwired: 2 in, 2 out]
                            n46 = property on="刷新图形" class="Bool (严格)"("Value"=TRUE ("刷新图形")) -> ()  [unwired: 2 in, 2 out]
                          }
                        }
                        n47 = Select(t=w112, s=w121, f=w123) -> (s? t:f=w122:string[])
                      }
                    }
                  }
                  frame True {
                    # "该参数已经注册在监控，本次添加无效"
                  }
                }
              }
            }
          }
          event "获取最后错误信息": Mouse Up {
            n48 = event-data() -> ()  [unwired: 1 in, 2 out]
            n49 = Initialize Array("a", 1024) -> (w133:string[])
            n50 = Concatenate Strings(w133) -> (w132:string)
            n51 = String Length(string=w132) -> (length=w131:i32)
            n52 = call <userlib>:"KLSL Get Last Err Info.vi"("error in (no error)"=w137, "nBuffLen"=w131, "szBuff"=w132) -> ("error out"=w136:errorcluster, "function return"=→"方法返回值":i32, "szBuff out"=→"返回的错误信息":string)  [unwired: 6 in]
          }
          event "获取仿真系统日志信息": Mouse Up {
            n53 = event-data() -> ()  [unwired: 1 in, 2 out]
            n54 = Initialize Array("a", 1024) -> (w149:string[])
            n55 = Concatenate Strings(w149) -> (w148:string)
            n56 = String Length(string=w148) -> (length=w147:i32)
            n57 = call <userlib>:"KLSL Get Simu Log Info.vi"("nLogLevel"=0, "nRemainLogCount"=300, "szLogInfo"=w148, "nLogBuffLen"=w147, "ulLogTime"=u32 0, "error in (no error)"=w153) -> ("nRemainLogCount out"=→"剩余日志条数":i32, "nLogLevel out"=→"返回的日志级别":i32, "szLogInfo out"=→"返回的日志信息":string, "function return"=→"方法返回值":i32, "error out"=w152:errorcluster)  [unwired: 4 in, 1 out]
          }
          event "参数": Double Click {
            n58 = event-data() -> ("CtlRef"=w165:refnum<vi>, "Row"=w159:i32)  [unwired: 1 in, 7 out]
            n59 = property class="MCListbox (严格)"(reference=w165) -> ("ItemNames"=w158:string[][])  [unwired: 1 in, 2 out]
            n60 = Array Size(array=w158) -> (size(s)=w162:i32[])
            n61 = Index Array(array=w162) -> (element=w161:i32)  [unwired: 1 in]
            n62 = Less Or Equal?(x=w159, y=w161) -> (x <= y?=w160:bool)
            n63 = case shown="真" w160 {
              tunnel: w159 -> [_ w177]
              tunnel: w158 -> [_ w176]
              tunnel: w157 -> [w166 w174]
              tunnel: [w166 w169] -> w156
              frame False {
              }
              frame True {
                n64 = Index Array(array=w176, index (row)=w177) -> (element=w175:string[])  [unwired: 1 in]
                n65 = Index Array(array=w175) -> (element #2=w168:string, element #3=w167:string)  [unwired: 3 in, 1 out]
                n66 = Decimal String To Number(string=w167) -> (number=w170:i32)  [unwired: 2 in, 1 out]
                n67 = call "set param.vi"("错误输入（无错误）"=w174, "数据大小in"=w170, "参数名in"=w168) -> ("错误输出"=w173:errorcluster, "数组out"=w171:dbl[], "确定"=w172:bool)  [unwired: 6 in]
                n68 = case shown="真" w172 {
                  tunnel: w173 -> [w178 w185]
                  tunnel: w171 -> [_ w179]
                  tunnel: w168 -> [_ w181]
                  tunnel: w170 -> [_ w182]
                  tunnel: [w178 w184] -> w169
                  frame False {
                  }
                  frame True {
                    n69 = call <userlib>:"KLSL Set Param Value.vi"("nDataSize"=w182, "error in (no error)"=w185, "pDataValue"=w179, "nOffSet"=0 ("nOffset"), "szParamName"=w181) -> ("error out"=w184:errorcluster, "function return"=w183:i32)  [unwired: 4 in, 1 out]
                    n70 = Equal To 0?(x=w183) -> (x = 0?=w189:bool)
                    n71 = Select(t="参数设置成功！", s=w189, f="参数设置失败！") -> (s? t:f=w188:string)
                    n72 = One Button Dialog(message=w188) -> ()  [unwired: 1 in, 1 out]
                  }
                }
              }
            }
          }
          event "加载": Value Change {
            n73 = event-data() -> ()  [unwired: 1 in, 6 out]
          }
          event "开始": Value Change {
            # "运行模型"
            n74 = event-data() -> ()  [unwired: 1 in, 6 out]
            n75 = call <userlib>:"KLSL Exec Project.vi"("error in (no error)"=w195) -> ("error out"=w194:errorcluster)  [unwired: 9 in, 1 out]
          }
          event "暂停": Value Change {
            # "暂停模型"
            n76 = event-data() -> ()  [unwired: 1 in, 6 out]
            n77 = call <userlib>:"KLSL Pause Project.vi"("error in (no error)"=w200) -> ("error out"=w199:errorcluster)  [unwired: 9 in, 1 out]
          }
          event "重置": Value Change {
            n78 = event-data() -> ()  [unwired: 1 in, 6 out]
            n79 = call <userlib>:"KLSL Stop Project.vi"("error in (no error)"=w209) -> ("error out"=w210:errorcluster, "function return"=w208:i32)  [unwired: 9 in]
            n80 = Equal To 0?(x=w208) -> (x = 0?=w207:bool)
            n81 = Select(t=string[] [], s=w207, f=w204) -> (s? t:f=w206:string[])
          }
          event "退出": Value Change {
            n82 = event-data() -> ()  [unwired: 1 in, 6 out]
          }
          event "获取工程状态": Mouse Up {
            n83 = event-data() -> ()  [unwired: 1 in, 2 out]
            n84 = Initialize Array("a", 1024) -> (w218:string[])
            n85 = Concatenate Strings(w218) -> (w217:string)
            n86 = String Length(string=w217) -> (length=w224:i32)
            n87 = call <userlib>:"KLSL Get Proj Simu Status.vi"("error in (no error)"=w226, "nProjStatus"=0, "nProjCfgBuffLen"=w224, "szProjCfg"=w217) -> ("error out"=w225:errorcluster, "nProjStatus out"=→"状态返回值":i32, "function return"=→"方法返回值":i32)  [unwired: 4 in, 1 out]
          }
          event "获取模型仿真状态": Mouse Up {
            n88 = event-data() -> ()  [unwired: 1 in, 2 out]
            n89 = Initialize Array ("初始化数组")(0.0, 4) -> (w233:dbl[])
            n90 = call <userlib>:"KLSL Get Model Simu Moni.vi"("nDataBuffLen"=4, "error in (no error)"=w239, "dMoniData"=w233, "nOverRunCount"=0, "szModelName"="模型名称输入框") -> ("error out"=w238:errorcluster, "dMoniData out"=→"dMoniData":dbl[], "nOverRunCount out"=→"超时返回值":i32, "function return"=→"方法返回值":i32)  [unwired: 3 in]
          }
          event "获取模型个数": Mouse Up {
            n91 = event-data() -> ()  [unwired: 1 in, 2 out]
            n92 = call <userlib>:"KLSL Get Proj Model Count.vi"("error in (no error)"=w245, "nCount"=0) -> ("error out"=w244:errorcluster, "nCount out"=→"模型个数":i32)  [unwired: 7 in, 1 out]
          }
          event "获取参数个数": Mouse Up {
            n93 = event-data() -> ()  [unwired: 1 in, 2 out]
            n94 = call <userlib>:"KLSL Get Proj Param Count.vi"("error in (no error)"=w251, "nCount"=0) -> ("error out"=w250:errorcluster, "nCount out"=→"参数个数":i32)  [unwired: 7 in, 1 out]
          }
          event "获取指定模型序号模型信息": Mouse Up {
            n95 = event-data() -> ()  [unwired: 1 in, 2 out]
            n96 = Initialize Array("a", 256) -> (w256:string[])
            n97 = Concatenate Strings(w256) -> (w255:string)
            n98 = String Length(string=w255) -> (length=w254:i32)
            n99 = call <userlib>:"KLSL Get Model Info.vi"("error in (no error)"=w263, "nNameBuffLen"=w254, "szModelName"=w255, "nModelIdx"="模型序号") -> ("error out"=w262:errorcluster, "szModelName out"=→"返回的模型信息":string, "function return"=→"方法返回值":i32)  [unwired: 5 in]
          }
          event "模型的下位机IP": Mouse Up {
            n100 = event-data() -> ()  [unwired: 1 in, 2 out]
            n101 = Initialize Array("a", 256) -> (w269:string[])
            n102 = Concatenate Strings(w269) -> (w268:string)
            n103 = String Length(string=w268) -> (length=w267:i32)
            n104 = call <userlib>:"KLSL Get Model Target.vi"("error in (no error)"=w274, "nTargetBuffLen"=w267, "szTargetIp"=w268, "szModelName"="模型名称") -> ("error out"=w273:errorcluster, "szTargetIp out"=→"返回的下位机IP":string)  [unwired: 5 in, 1 out]
          }
          event "模型名称获取ID": Mouse Up {
            n105 = event-data() -> ()  [unwired: 1 in, 2 out]
            n106 = call <userlib>:"KLSL Get Model Id By Name.vi"("error in (no error)"=w282, "nModelId"=0, "szModelName"="模型名称") -> ("error out"=w281:errorcluster, "nModelId out"=→"返回模型ID":i32, "function return"=→"方法返回值":i32)  [unwired: 6 in]
          }
          event "获取参数ID通过名称": Mouse Up {
            n107 = event-data() -> ()  [unwired: 1 in, 2 out]
            n108 = call <userlib>:"KLSL Get Param Id By Name.vi"("error in (no error)"=w290, "nParamId"=0, "szParamName"="参数名称") -> ("error out"=w289:errorcluster, "nParamId out"=→"返回参数ID":i32, "function return"=→"方法返回值":i32)  [unwired: 6 in]
          }
          event "根据参数名称获取模型名称": Mouse Up {
            n109 = event-data() -> ()  [unwired: 1 in, 2 out]
            n110 = Initialize Array("a", 1024) -> (w295:string[])
            n111 = Concatenate Strings(w295) -> (w294:string)
            n112 = String Length(string=w294) -> (length=w293:i32)
            n113 = call <userlib>:"KLSL Get Model Name By Param Name.vi"("error in (no error)"=w302, "nNameBuffLen"=w293, "szModelName"=w294, "szParamName"="参数名称") -> ("error out"=w301:errorcluster, "szModelName out"=→"模型名称":string, "function return"=→"方法返回值":i32)  [unwired: 5 in]
          }
          event "获取信号值": Mouse Up {
            w305 = 1024
            n114 = event-data() -> ()  [unwired: 1 in, 2 out]
            n115 = Initialize Array(0.0, w305) -> (w309:dbl[])
            n116 = call <userlib>:"KLSL Get Out Sig Value.vi"("nDataBuffLen"=w305, "error in (no error)"=w313, "pDataValue"=w309, "nOffSet"="数组偏移量", "szOutSigName"="信号名称") -> ("error out"=w312:errorcluster, "pDataValue out"=→"pData":dbl[], "function return"=→"方法返回值":i32)  [unwired: 3 in, 1 out]
          }
          event "注册参数瞬态": Mouse Up {
            n117 = event-data() -> ()  [unwired: 1 in, 2 out]
            n118 = call <userlib>:"KLSL Reg Param Latest Value.vi"("error in (no error)"=w319, "nOffSet"="数组偏移", "szParamName"="参数名称") -> ("error out"=w317:errorcluster, "function return"=→"注册参数瞬态返回值":i32)  [unwired: 7 in]
          }
          event "获取参数值瞬态": Mouse Up {
            w323 = 1024
            n119 = event-data() -> ()  [unwired: 1 in, 2 out]
            n120 = Initialize Array(0.0, w323) -> (w330:dbl[])
            n121 = call <userlib>:"KLSL Get Param Latest Value.vi"("szParamName"="参数名称", "nDataBuffLen"=w323, "nOffSet"="数组偏移", "pTimeOffset"=0.0, "pDataValue"=w330, "error in (no error)"=w335, "nFactDataLen"=0) -> ("function return"=→"获取参数值瞬态返回值":i32, "pTimeOffset out"=→"时间偏移返回值":dbl, "pDataValue out"=→"pDataValue out":dbl[], "nFactDataLen out"=→"实际有效数据长度":i32, "error out"=w334:errorcluster)  [unwired: 4 in]
          }
          event "获取参数值连续": Mouse Up {
            w343 = 1024
            n122 = event-data() -> ()  [unwired: 1 in, 2 out]
            n123 = Initialize Array(0.0, w343) -> (w344:dbl[])
            n124 = call <userlib>:"KLSL Get Param Period Value.vi"("szParamName"="参数名称", "pDataValue"=w344, "nFactDataLen"=100, "nOffSet"="数组偏移", "nSampleUs"=1, "pTimeOffset"=w344, "error in (no error)"=w350, "nDataBuffLen"=w343) -> ("pDataValue out"=→"返回的参数值":dbl[], "nFactDataLen out"=→"实际有效数据长度":i32, "function return"=→"获取参数值连续返回值":i32, "pTimeOffset out"=→"返回的时间偏移":dbl[], "error out"=w349:errorcluster)  [unwired: 3 in]
          }
          event "注销参数瞬态": Mouse Up {
            n125 = event-data() -> ()  [unwired: 1 in, 2 out]
            n126 = call <userlib>:"KLSL Un Param Latest Value.vi"("error in (no error)"=w357, "nOffSet"="数组偏移", "szParamName"="参数名称") -> ("error out"=w356:errorcluster, "function return"=→"注销参数瞬态返回值":i32)  [unwired: 7 in]
          }
          event "注册参数连续": Mouse Up {
            n127 = event-data() -> ()  [unwired: 1 in, 2 out]
            n128 = call <userlib>:"KLSL Reg Param Period Value.vi"("nCachedDataCount"=200, "error in (no error)"=w366, "nSampleUs"=1, "nOffSet"="数组偏移", "szParamName"="参数名称") -> ("error out"=w365:errorcluster, "function return"=→"注册参数连续返回值":i32)  [unwired: 5 in]
          }
          event "注销连续": Mouse Up {
            n129 = event-data() -> ()  [unwired: 1 in, 2 out]
            n130 = call <userlib>:"KLSL Un Reg Param Period Value.vi"("error in (no error)"=w374, "nSampleUs"=1, "nOffSet"="数组偏移", "szParamName"="参数名称") -> ("error out"=w373:errorcluster, "function return"=→"注销连续返回值":i32)  [unwired: 6 in]
          }
          event "获取参数值": Mouse Up {
            w378 = 1024
            n131 = event-data() -> ()  [unwired: 1 in, 2 out]
            n132 = Initialize Array(0.0, w378) -> (w381:dbl[])
            n133 = call <userlib>:"KLSL Get Param Value.vi"("nDataBuffLen"=w378, "error in (no error)"=w385, "pDataValue"=w381, "nOffSet"="数组偏移量", "szParamName"="参数名称") -> ("error out"=w384:errorcluster, "pDataValue out"=→"pData":dbl[], "function return"=→"方法返回值":i32)  [unwired: 3 in, 1 out]
          }
          event "注册输出信号瞬态": Mouse Up {
            n134 = event-data() -> ()  [unwired: 1 in, 2 out]
            n135 = call <userlib>:"KLSL Reg Out Sig Latest Value.vi"("error in (no error)"=w392, "nOffSet"="数组偏移", "szOutSigName"="输出信号名称") -> ("error out"=w391:errorcluster, "function return"=→"注册输出信号瞬态返回值":i32)  [unwired: 7 in]
          }
          event "获取信号值瞬态": Mouse Up {
            w400 = 1024
            n136 = event-data() -> ()  [unwired: 1 in, 2 out]
            n137 = Initialize Array(0.0, w400) -> (w401:dbl[])
            n138 = call <userlib>:"KLSL Get Out Sig Latest Value.vi"("szOutSigName"="信号名称", "nDataBuffLen"=w400, "nOffSet"="数组偏移", "pTimeOffset"=0.0, "pDataValue"=w401, "error in (no error)"=w407, "nFactDataLen"=0) -> ("function return"=→"信瞬方法返回值":i32, "pTimeOffset out"=→"时间偏移返回值":dbl, "pDataValue out"=→"返回的信号值":dbl[], "nFactDataLen out"=→"实际有效数据长度":i32, "error out"=w406:errorcluster)  [unwired: 4 in]
          }
          event "注销输出信号瞬态": Mouse Up {
            n139 = event-data() -> ()  [unwired: 1 in, 2 out]
            n140 = call <userlib>:"KLSL Un Reg Out Sig Latest Value.vi"("error in (no error)"=w414, "nOffSet"="数组偏移", "szOutSigName"="输出信号名称") -> ("error out"=w413:errorcluster, "function return"=→"注销输出信号瞬态返回值":i32)  [unwired: 7 in]
          }
          event "注册输出信号连续": Mouse Up {
            n141 = event-data() -> ()  [unwired: 1 in, 2 out]
            n142 = call <userlib>:"KLSL Reg Out Sig Period Value.vi"("nCachedDataCount"=100, "error in (no error)"=w423, "nSampleUs"=1, "nOffSet"="数组偏移", "szOutSigName"="输出信号名称") -> ("error out"=w422:errorcluster, "function return"=→"注册输出信号连续返回值":i32)  [unwired: 5 in]
          }
          event "获取信号值连续": Mouse Up {
            w426 = 1024
            n143 = event-data() -> ()  [unwired: 1 in, 2 out]
            n144 = Initialize Array(0.0, w426) -> (w432:dbl[])
            n145 = call <userlib>:"KLSL Get Out Sig Period Value.vi"("szOutSigName"="信号名称", "pDataValue"=w432, "nFactDataLen"=0, "nOffSet"="数组偏移", "nSampleUs"=1, "pTimeOffset"=w432, "error in (no error)"=w438, "nDataBuffLen"=w426) -> ("pDataValue out"=→"信号连续返回值":dbl[], "nFactDataLen out"=→"实际有效数据长度":i32, "function return"=→"信连方法返回值":i32, "pTimeOffset out"=→"pTimeOffset out":dbl[], "error out"=w437:errorcluster)  [unwired: 3 in]
          }
          event "注销输出信号连续": Mouse Up {
            n146 = event-data() -> ()  [unwired: 1 in, 2 out]
            n147 = call <userlib>:"KLSL Un Reg Out Sig Period Value.vi"("error in (no error)"=w446, "nSampleUs"=1, "nOffSet"="数组偏移", "szOutSigName"="输出信号名称") -> ("error out"=w445:errorcluster, "function return"=→"注销输出信号连续返回值":i32)  [unwired: 6 in]
          }
          event "注册录制组": Mouse Up {
            n148 = event-data() -> ()  [unwired: 1 in, 2 out]
            n149 = call <userlib>:"KLSL Reg Record Group.vi"("szGroupName"="录制组名称", "szFileDir"="存储文件的路径", "nOutSigParamIdList"="参数/输出信号ID列表", "nListLen"="列表长度", "nSampleUs"="采样率", "dRecordTimeSec"="录制时长", "nDataFormat"="数据格式", "error in (no error)"=w463, "szFileName"="录制文件名", "nOutSigParamOffsetList"="参数输出信号偏移") -> ("nOutSigParamIdList out"=→"nOutSigParamIdList out":i32[], "nOutSigParamOffsetList out"=→"nOutSigParamOffsetList out":i32[], "function return"=→"function return":i32, "error out"=w451:errorcluster)  [unwired: 2 in]
            n150 = disable-structure shown="禁用" {
              disable-tunnel: w451 -> [w468 _]
              disable-tunnel: [w467 _] -> w450
              disable-tunnel: "录制组名称" -> [w466 _]
              frame Disabled {
                n151 = while {
                  shift-right: [w474] -> w467
                  shift-left: w468 -> [w475]
                  tunnel: w466 -> [w473]
                  stop <- w469 stop-if-true
                  n152 = call <userlib>:"KLSL Get Record Group Status.vi"("error in (no error)"=w475, "nStatus"=0, "szGroupName"=w473) -> ("error out"=w474:errorcluster, "nStatus out"=w471:i32)  [unwired: 6 in, 1 out]
                  "nStatus out" <- w471
                  n153 = Equal?(x=w471, y=4) -> (x = y?=w469:bool)
                }
              }
              frame Enabled {
              }
            }
          }
          event "获取录制组状态": Mouse Up {
            n154 = event-data() -> ()  [unwired: 1 in, 2 out]
            n155 = call <userlib>:"KLSL Get Record Group Status.vi"("error in (no error)"=w481, "nStatus"=4, "szGroupName"="录制组名称") -> ("error out"=w480:errorcluster, "nStatus out"=→"录制组状态":i32, "function return"=→"方法返回值":i32)  [unwired: 6 in]
          }
          event "注销录制组": Mouse Up {
            n156 = event-data() -> ()  [unwired: 1 in, 2 out]
            n157 = call <userlib>:"KLSL Un Reg Record Group.vi"("error in (no error)"=w487, "szGroupName"="录制组名称") -> ("error out"=w486:errorcluster, "function return"=→"方法返回值":i32)  [unwired: 8 in]
          }
          event "获取信号ID通过名称": Mouse Up {
            n158 = event-data() -> ()  [unwired: 1 in, 2 out]
            n159 = call <userlib>:"KLSL Get Out Sig Id By Name.vi"("error in (no error)"=w495, "nOutSigId"=0, "szOutSigName"="信号名称") -> ("error out"=w494:errorcluster, "nOutSigId out"=→"返回信号ID":i32, "function return"=→"方法返回值":i32)  [unwired: 6 in]
          }
        }
      }
      frame "initial" {
        w499 = string[][] [] ("项名")
        w498 = FALSE ("初始化状态")
        # "初始化所有界面控件"
        n160 = for {
          tunnel: w509 -> [w512] mode=indexing
          n161 = property class="Bool"(reference=w512, "DisabledEnum"=T4."Disabled and Grayed Out" ("禁用")) -> ()  [unwired: 1 in, 2 out]
        }
        n162 = property on="连接" class="Bool"("DisabledEnum"=T4."Enabled" ("禁用")) -> ()  [unwired: 2 in, 2 out]
        n163 = property on="信号" class="MCListbox (严格)"("ItemNames"=w499) -> (error out=w506:errorcluster)  [unwired: 2 in, 1 out]
        n164 = property on="参数" class="MCListbox (严格)"(error in=w506, "ItemNames"=w499) -> (error out=w500:errorcluster)  [unwired: 1 in, 1 out]
        n165 = property on="XY Graph" class="XYGraph (严格)"("Caption.Text"="信号波形图" ("标题.文本")) -> ()  [unwired: 2 in, 2 out]
        n166 = property on="信号1" class="MCListbox (严格)"(error in=w500, "ItemNames"=w499) -> ()  [unwired: 1 in, 2 out]
        n167 = property on="连接状态" class="Bool (严格)"("Value"=w498) -> ()  [unwired: 2 in, 2 out]
        n168 = property on="加载状态" class="Bool (严格)"("Value"=w498) -> ()  [unwired: 2 in, 2 out]
        n169 = property on="刷新图形" class="Bool (严格)"("Value"=FALSE ("刷新图形")) -> ()  [unwired: 2 in, 2 out]
        n170 = local write "列表已更新"(FALSE ("更新信号和参数列表")) -> ()
      }
      frame "connect target" {
        n171 = case shown="真" "连接" {
          tunnel: w520 -> [w522 w527]
          tunnel: [w522 w526] -> w513
          tunnel: [_ w523] -> w518
          frame False {
          }
          frame True {
            n172 = call <userlib>:"KLSL Create Connect.vi"("error in (no error)"=w527, "szCtrlIp"="仿真系统上位机IP地址") -> ("error out"=w526:errorcluster, "function return"=w525:i32)  [unwired: 8 in]
            "连接返回值" <- w525
            n173 = Equal To 0?(x=w525) -> (x = 0?=w523:bool)
            "连接状态" <- w523
            n174 = Select(t=T4."Disabled and Grayed Out" ("禁用"), s=w523, f=T4."Enabled") -> (s? t:f=w528:T4)
            n175 = property on="连接" class="Bool"("DisabledEnum"=w528) -> ()  [unwired: 2 in, 2 out]
          }
        }
        n176 = Select(t=T3."get state", s=w518, f=T3."connect target") -> (s? t:f=w517:T3)
      }
      frame "get state" {
        # "获取工程的最新状态"
        n177 = call <userlib>:"KLSL Get Proj Simu Status.vi"("error in (no error)"=w534, "nProjStatus"=0, "nProjCfgBuffLen"=256) -> ("error out"=w532:errorcluster, "nProjStatus out"=w536:i32, "function return"=w537:i32)  [unwired: 5 in, 1 out]
        n178 = case shown="0" w537 {
          tunnel: w536 -> [w557 _]
          tunnel: w540 -> [_ w562]
          tunnel: [w556 w562] -> w533
          frame 0 {
            # "获取状态成功"
            n179 = case shown="0, 默认" w557 {
              tunnel: [enum16{"未加载", "运行中", "暂停中"}."未加载" enum16{"未加载", "运行中", "暂停中"}."未加载" enum16{"未加载", "运行中", "暂停中"}."暂停中" enum16{"未加载", "运行中", "暂停中"}."运行中"] -> w556
              frame 0, Default {
              }
              frame 1 {
              }
              frame 2 {
              }
              frame 3 {
              }
            }
          }
          frame 1, Default {
            # "获取状态失败"
          }
        }
        n180 = case shown="\"运行中\", 默认" w533 {
          tunnel: w532 -> [w543 w544]
          tunnel: [w543 w546] -> w531
          frame "未加载" {
            n181 = local write "列表已更新"(FALSE ("列表已更新")) -> ()
          }
          frame "运行中", Default {
            n182 = local read "列表已更新"() -> (w545:bool)
            n183 = case shown="假" w545 {
              tunnel: [w550 w555] -> w546
              tunnel: w544 -> [_ w555]
              frame False {
                n184 = call "get sig info.vi"() -> ("错误输出"=w554:errorcluster, "信号列表"=w552:string[][])  [unwired: 10 in]
                n185 = property on="信号" class="MCListbox (严格)"("ItemNames"=w552) -> ()  [unwired: 2 in, 2 out]
                n186 = call "get param info.vi"("错误输入（无错误）"=w554) -> ("错误输出"=w549:errorcluster, "参数列表"=w553:string[][])  [unwired: 9 in]
                n187 = property on="参数" class="MCListbox (严格)"("ItemNames"=w553) -> ()  [unwired: 2 in, 2 out]
                n188 = call "get sig info2.vi"("错误输入（无错误）"=w549) -> ("错误输出"=w548:errorcluster, "信号列表1"=w547:string[][])  [unwired: 9 in]
                n189 = property on="信号1" class="MCListbox (严格)"("ItemNames"=w547) -> ()  [unwired: 2 in, 2 out]
                n190 = property on="列表已更新" class="Bool (严格)"(error in=w548, "Value"=TRUE ("列表已更新")) -> (error out=w550:errorcluster)  [unwired: 1 in, 1 out]
              }
              frame True {
              }
            }
          }
        }
      }
      frame "load project" {
        n191 = Path To String(path="工程配置文件") -> (string=w566:string)
        n192 = call <userlib>:"KLSL Load Project.vi"("error in (no error)"=w565, "szProjCfg"=w566) -> ("error out"=w563:errorcluster, "function return"=w564:i32)  [unwired: 8 in]
        "加载返回值" <- w564
        n193 = Equal To 0?(x=w564) -> (x = 0?=→"加载状态":bool)
      }
      frame "monitoring" {
        n194 = Array Size(array=w578) -> (size(s)=w581:i32)
        n195 = Equal?(x=w581, y=0) -> (x = y?=w579:bool)
        n196 = case shown="假" w579 {
          tunnel: w582 -> [w611 w615]
          tunnel: [w610 w615] -> w575
          tunnel: w578 -> [w612 w614]
          tunnel: [w612 w614] -> w577
          frame False {
            w585 = dbl[] []
            # "有新信号注册，刷新图形"
            # "图形缓存大小，默认1024"
            n197 = property on="缓冲示波个数" class="DigNum (严格)"() -> ("Value"=w607:i32)  [unwired: 2 in, 2 out]
            n198 = Index Array(array=w612) -> (element #2=w608:string, element #4=w604:string)  [unwired: 4 in, 2 out]
            n199 = Decimal String To Number(string=w604) -> (number=w603:i32)  [unwired: 2 in, 1 out]
            n200 = Initialize Array(0.0 ("数值"), w607) -> (w609:dbl[])
            n201 = call <userlib>:"KLSL Get Out Sig Period Value.vi"("szOutSigName"=w608, "pDataValue"=w609, "nFactDataLen"=0, "nOffSet"=w603, "nSampleUs"=1, "pTimeOffset"=w609, "error in (no error)"=w611, "nDataBuffLen"=w607) -> ("pDataValue out"=w601:dbl[], "nFactDataLen out"=w599:i32, "pTimeOffset out"=w600:dbl[], "error out"=w610:errorcluster)  [unwired: 3 in, 1 out]
            n202 = Array Subset(array=w601, length=w599) -> (w596:dbl[])  [unwired: 1 in]
            n203 = Array Subset(array=w600, length=w599) -> (w595:dbl[])  [unwired: 1 in]
            n204 = feedback #1(dbl[] []) -> (w598:dbl[])
            n205 = Build Array (concatenate)(w598, w596) -> (w584:dbl[])
            n206 = feedback #2(dbl[] []) -> (w594:dbl[])
            n207 = Build Array (concatenate)(w594, w595) -> (w587:dbl[])
            n208 = Array Size(array=w587) -> (size(s)=w591:i32)
            n209 = Greater?(x=w591, y="缓冲点数") -> (0:w589:bool)
            n210 = Or(x=w589, y="刷新图形") -> (x .or. y?=w586:bool)
            n211 = Select(t=w585, s=w586, f=w587) -> (s? t:f=w588:dbl[])
            n212 = feedback-in #2(w588) -> ()
            n213 = Select(t=w585, s=w586, f=w584) -> (s? t:f=w583:dbl[])
            n214 = feedback-in #1(w583) -> ()
            n215 = Bundle(w588, w583) -> (→"XY Graph":cluster{dbl[], dbl[]})  [unwired: 1 in]
          }
          frame True {
          }
        }
        n216 = property on="刷新图形" class="Bool (严格)"(error in=w575, "Value"=FALSE ("刷新图形")) -> (error out=w574:errorcluster)  [unwired: 1 in, 1 out]
      }
      frame "exit" {
        # "退出时不改变当前模型的状态"
        n217 = call <userlib>:"KLSL Dis Connect.vi"("error in (no error)"=w618) -> ("error out"=w617:errorcluster, "function return"=→"function return 2":i32)  [unwired: 9 in]
      }
      frame "error" {
        w626 = T6 4 items=["无对话框", "确定信息", "继续或停止信息", "确定信息＋警告", "继续/停止+警告"] ("type of dialog (OK msg:1)")
        n218 = call <vilib>:"General Error Handler.vi"("type of dialog (OK msg:1)"=w626, "error in (no error)"=w627) -> ("error out"=w625:errorcluster)  [unwired: 9 in, 4 out]
      }
    }
    n219 = Select(t=T3."error", s=w21, f=w20) -> (s? t:f=w19:T3)
    n220 = Select(t=T3."exit", s="退出", f=w19) -> (s? t:f=w16:T3)
  }
  n221 = disable-structure shown="RUN_TIME_ENGINE==True" {
    disable-tunnel: w2 -> [_ _]
    frame condition #0 (active) {
    }
    frame condition #1 {
      n222 = Quit LabVIEW(quit? (T)=TRUE ("退出？(T)")) -> ()
    }
  }
